vi "New__slk_tc.vi"(0 "tree refnum":refnum<vi>, 11 "error in (no error)":errorcluster) -> (4 "tree control out":refnum<class "TreeControl.lvclass">, 15 "error out":errorcluster)   [LabVIEW 2020, in "TreeControl.lvclass"]
doc: "Creats a new TREE CONTROL object."
uses:
  Library/TreeControl.lvclass
  Library/TreeControl.lvclass/TreeControl.ctl
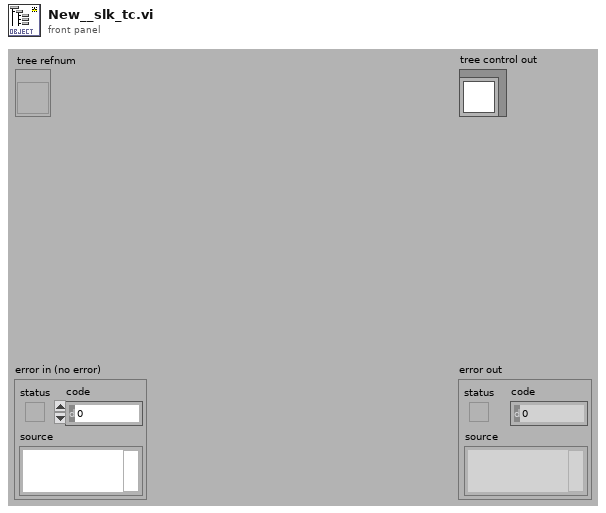
[diagram p1: front panel]
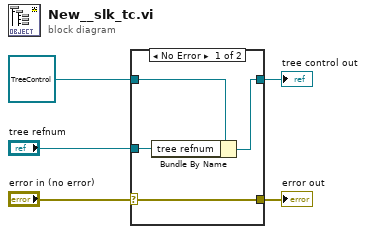
[diagram p0: block diagram]
diagram:
  n1 = case shown="No Error" "error in (no error)" {
    selector: "error in (no error)" -> [w8 w11]
    tunnel: [w8 w11] -> w4
    tunnel: [w7 w10] -> w2
    tunnel: refnum<class "TreeControl.lvclass"> refnum ("Tree Control in") -> [w9 w10]
    tunnel: "tree refnum" -> [w6 _]
    frame No Error {
      n2 = Bundle By Name(cluster=w9, "tree refnum"=w6) -> (w7:refnum<class "TreeControl.lvclass">)
    }
    frame Error {
    }
  }
  "error out" <- w4
  "tree control out" <- w2
